vi "Test Create and Compose.vi"() -> ()   [LabVIEW 2011]
uses:
  Orient3d Class.lvclass
  Vec3d Class/Vec3d Class.lvclass
panel:
  out "Net Orient":cluster{"x":dbl, "y":dbl, "z":dbl, "w":dbl}
  in  "Orient2":cluster{"x":dbl, "y":dbl, "z":dbl, "w":dbl}
  in  "Orient1":cluster{"x":dbl, "y":dbl, "z":dbl, "w":dbl}
  out "Rotated x-hat Vector":cluster{"X":dbl, "Y":dbl, "Z":dbl}
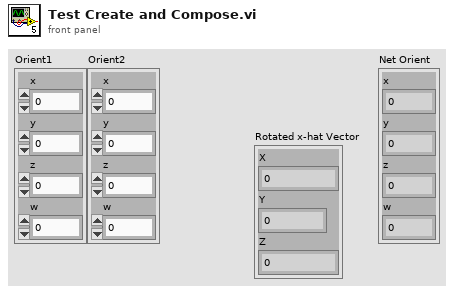
[diagram p1: front panel]
types:
  T1 = typedef "Quaternion.ctl" = cluster{"x":dbl, "y":dbl, "z":dbl, "w":dbl}
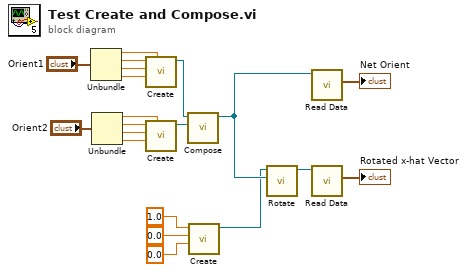
[diagram p0: block diagram]
diagram:
  n1 = Unbundle("Orient1") -> ("x"=w4:dbl, "y"=w3:dbl, "z"=w2:dbl, "w"=w1:dbl)
  n2 = Unbundle("Orient2") -> ("x"=w8:dbl, "y"=w7:dbl, "z"=w6:dbl, "w"=w5:dbl)
  n3 = call "Create.vi"("x"=w4, "w"=w1, "z"=w2, "y"=w3) -> ("Orient3d out"=w20:refnum<class "Orient3d Class.lvclass">)  [unwired: 6 in, 1 out]
  n4 = call "Create.vi"("x"=w8, "w"=w5, "z"=w6, "y"=w7) -> ("Orient3d out"=w19:refnum<class "Orient3d Class.lvclass">)  [unwired: 6 in, 1 out]
  n5 = call "Compose.vi"("Orient3d 2"=w19, "Orient3d 1"=w20) -> ("Orient3d out"=w15:refnum<class "Orient3d Class.lvclass">)  [unwired: 8 in, 1 out]
  n6 = call "Create.vi"("Z"=0.0 ("Y"), "Y"=0.0, "X"=1.0) -> ("Vec3d Class out"=w14:refnum<class "Vec3d Class.lvclass">)  [unwired: 7 in, 1 out]
  n7 = call "Rotate.vi"("Orient3d in"=w15, "Vec3d in"=w14) -> ("Vec3d out"=w13:refnum<class "Vec3d Class.lvclass">)  [unwired: 8 in, 1 out]
  n8 = call "Read Data.vi"("Orient3d in"=w15) -> ("Quaternion"=→"Net Orient":T1)  [unwired: 8 in, 2 out]
  n9 = call-dynamic "Read Data.vi"("Vec3d Class in"=w13) -> ("Data"=→"Rotated x-hat Vector":cluster{"X":dbl, "Y":dbl, "Z":dbl})  [unwired: 8 in, 2 out]
